vi "Overall Example.vi"() -> ()   [LabVIEW 2022 SP3]
uses:
  <instrlib>/openDAQ/Public/Classes/IInstance/IInstance.lvclass
  C:/Program Files (x86)/National Instruments/LabVIEW 2022/instr.lib/openDAQ/Public/Classes/IDevice/IDevice.lvclass
  C:/Program Files (x86)/National Instruments/LabVIEW 2022/instr.lib/openDAQ/Public/Classes/IComponent/IComponent.lvclass
  <instrlib>/openDAQ/Public/Classes/IComponent/IComponent.lvclass
  <instrlib>/openDAQ/Public/Classes/ISignal/ISignal.lvclass
  <instrlib>/openDAQ/Public/Classes/daqUtils/daqUtils.lvlib
  <instrlib>/openDAQ/Public/Classes/IDevice/IDevice.lvclass
panel:
  in  "btn:streamReader":bool
  in  "btn:multiReader":bool
  in  "btn:configureDevice":bool
  in  "Available Signals":i32[](listbox)
  in  "Btn:Stop":bool
  in  "MCL:available Devices":i32(listbox) caption="Available Devices"
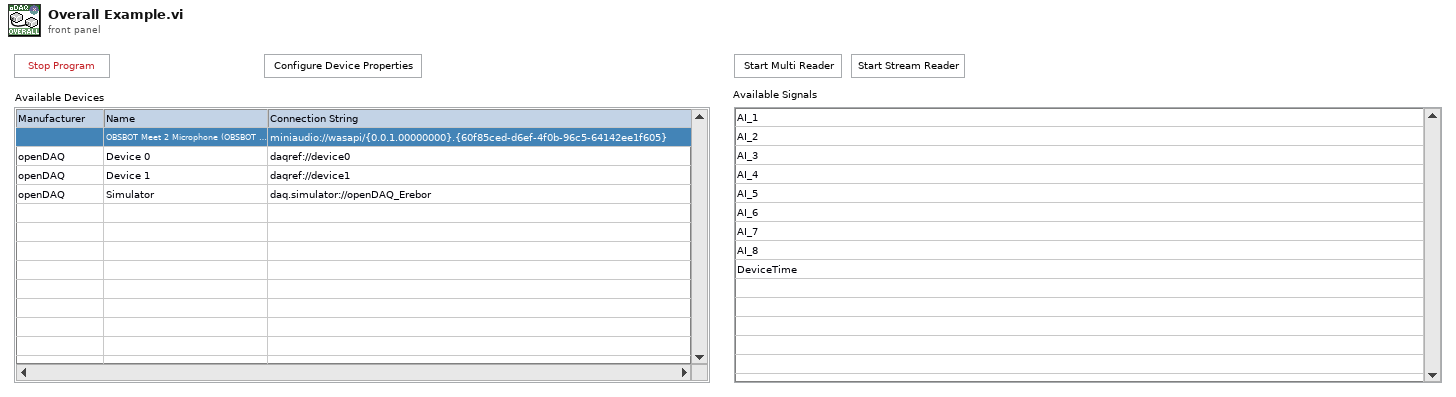
[diagram p1: front panel]
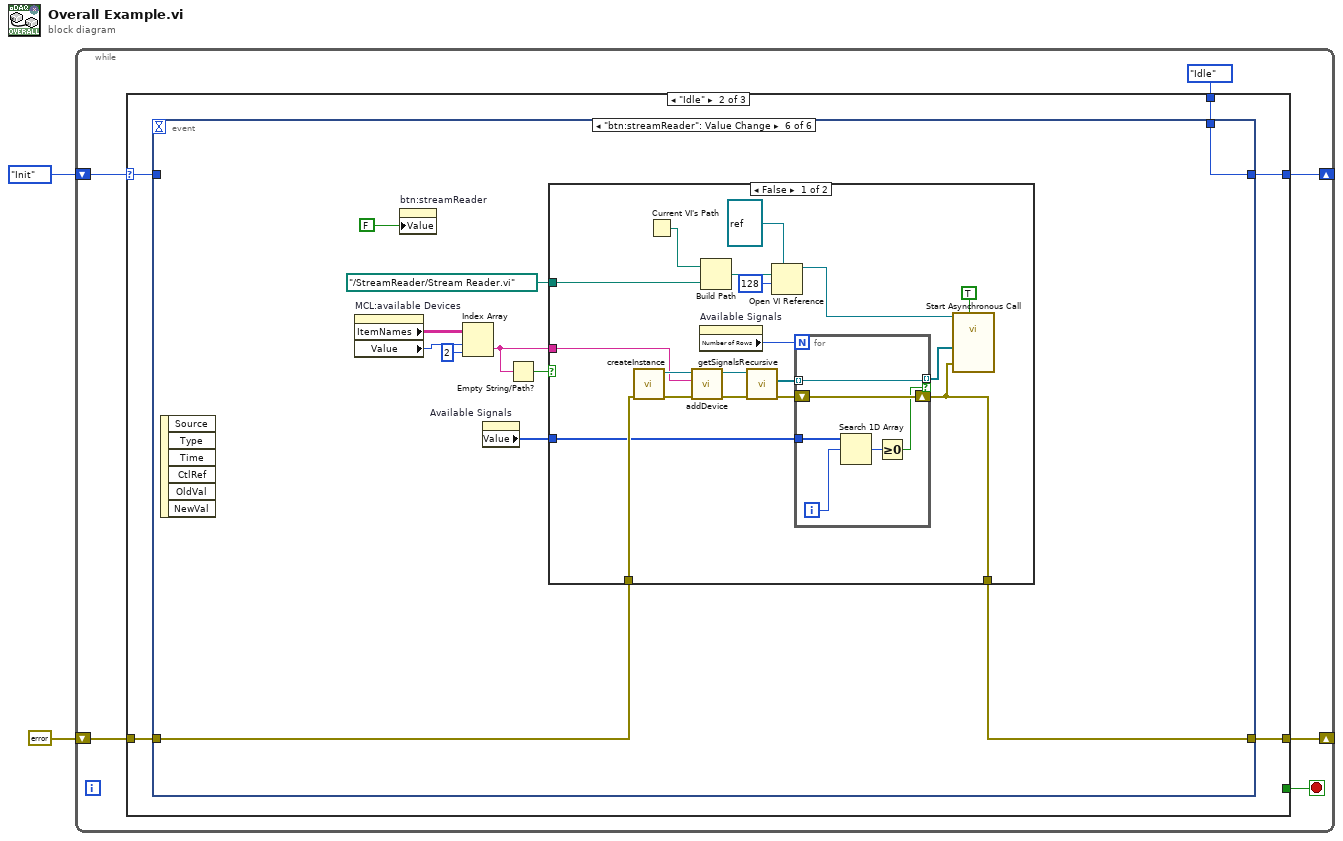
[diagram p0: block diagram]
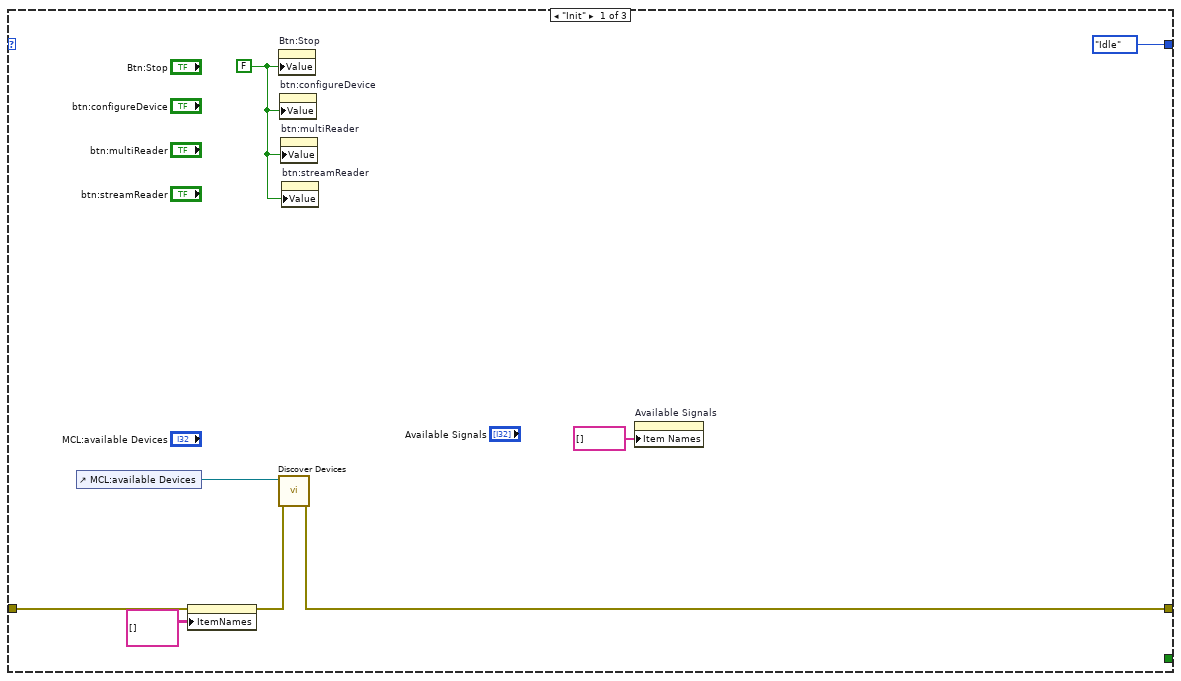
[diagram p2: hidden frame]
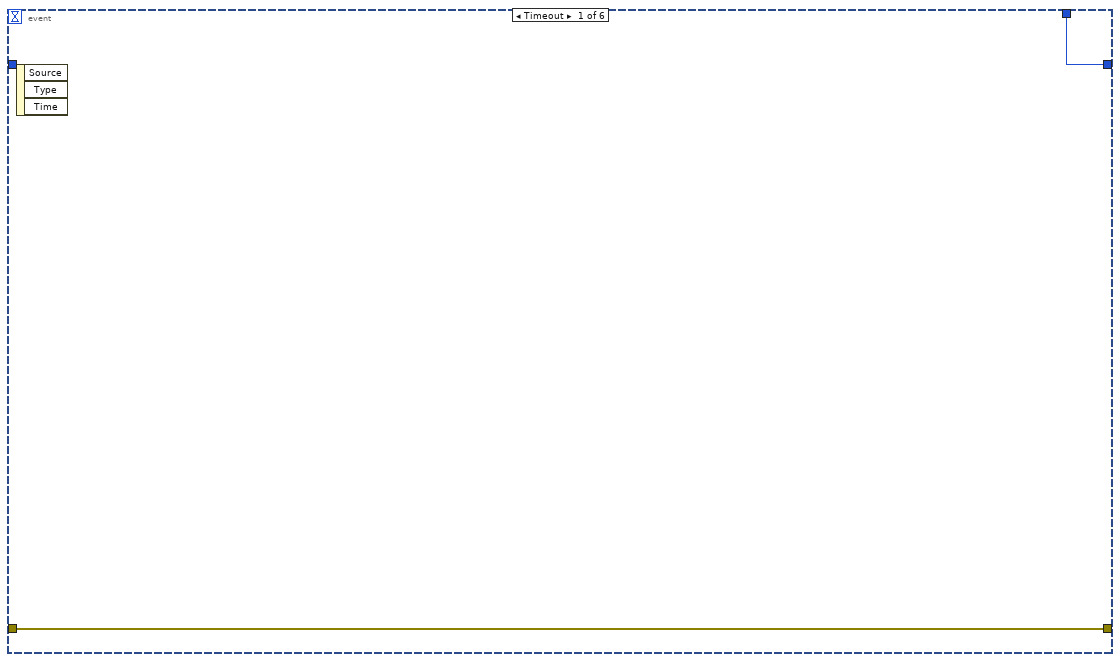
[diagram p3: hidden frame]
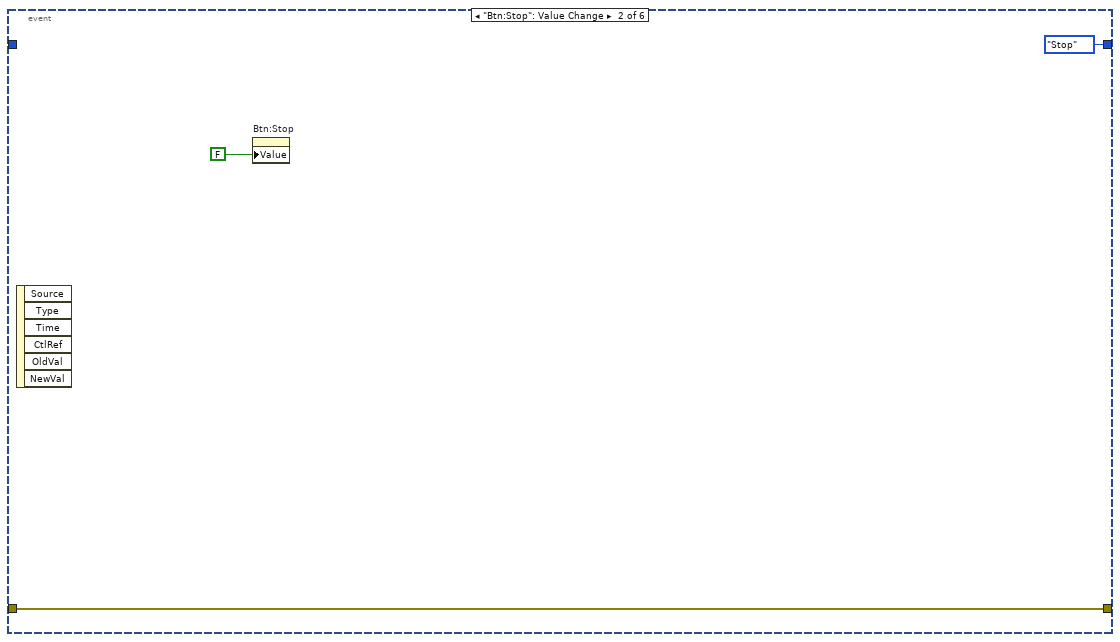
[diagram p4: hidden frame]
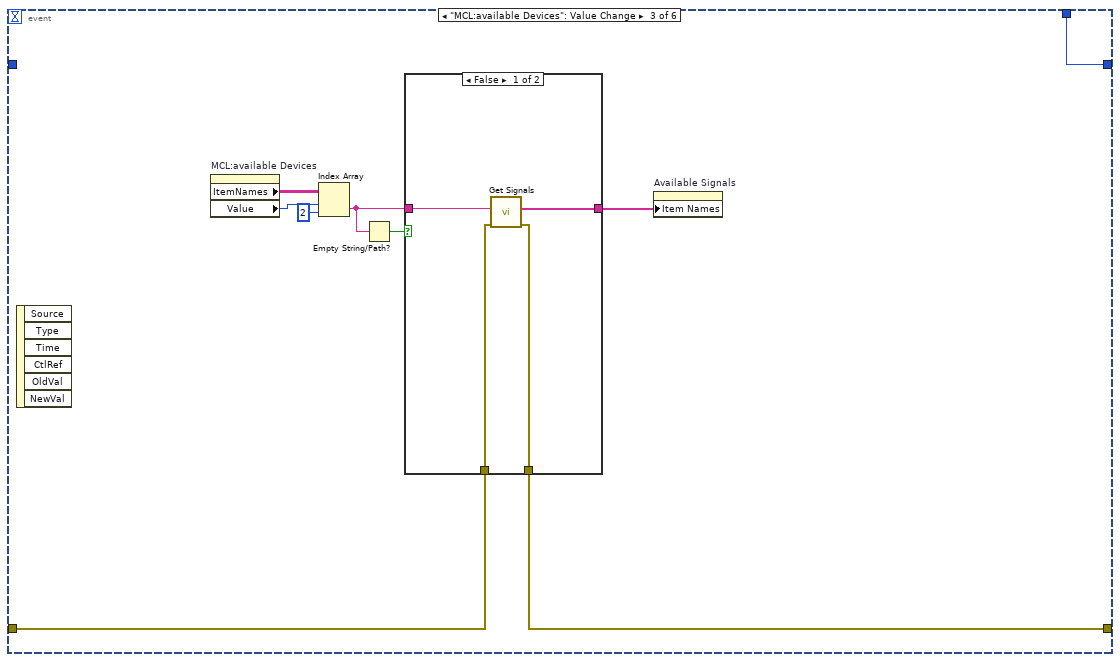
[diagram p5: hidden frame]
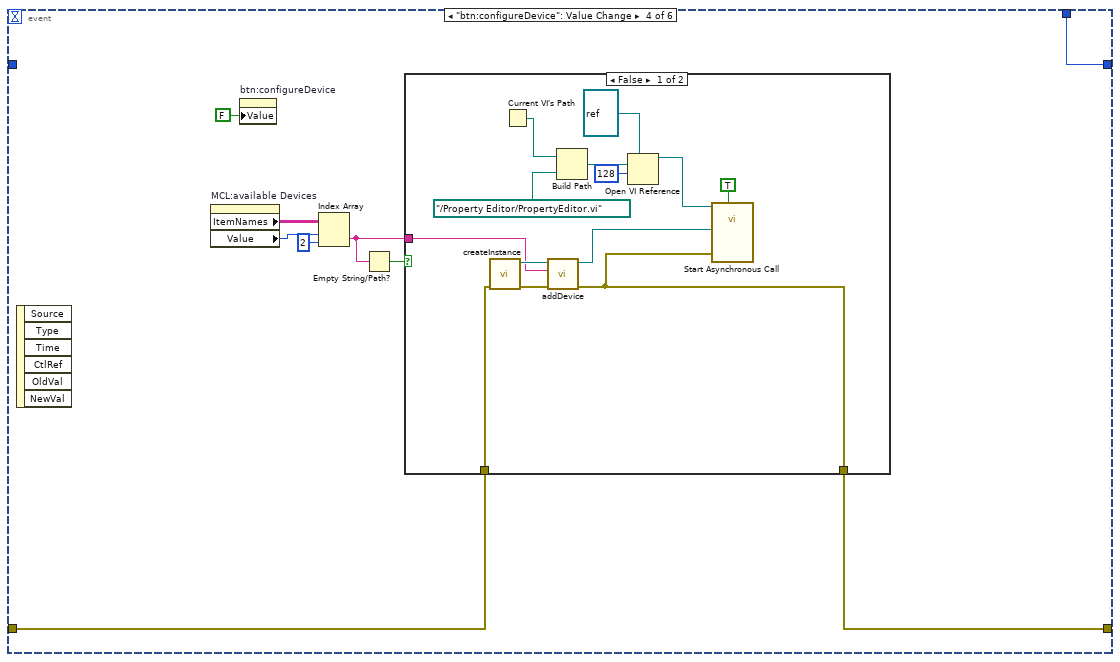
[diagram p7: hidden frame]
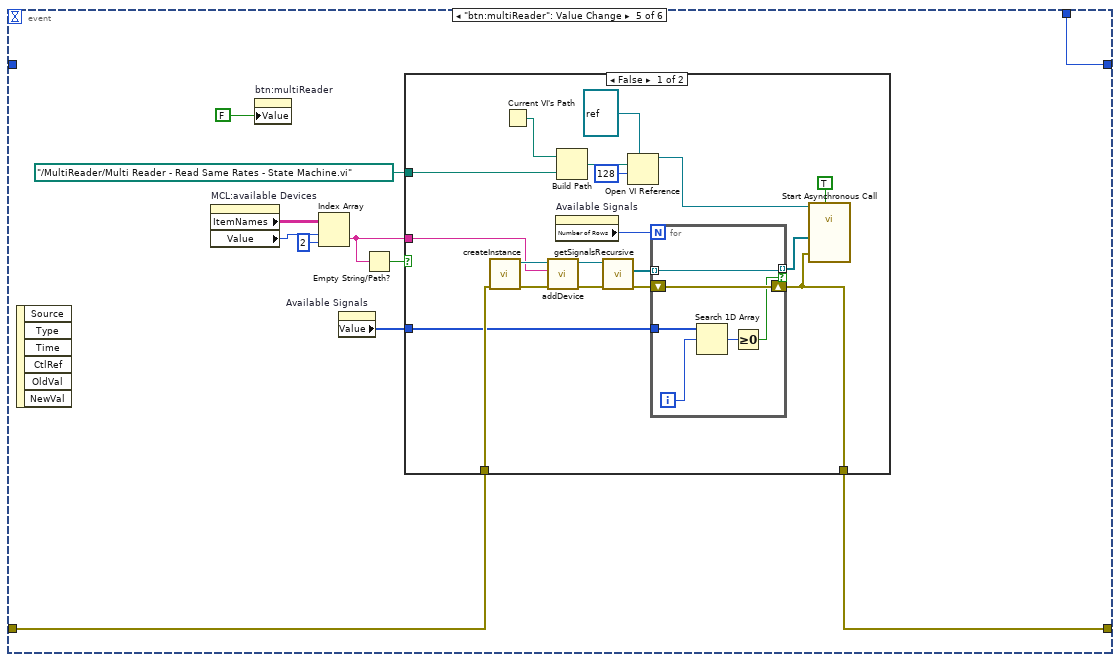
[diagram p9: hidden frame]
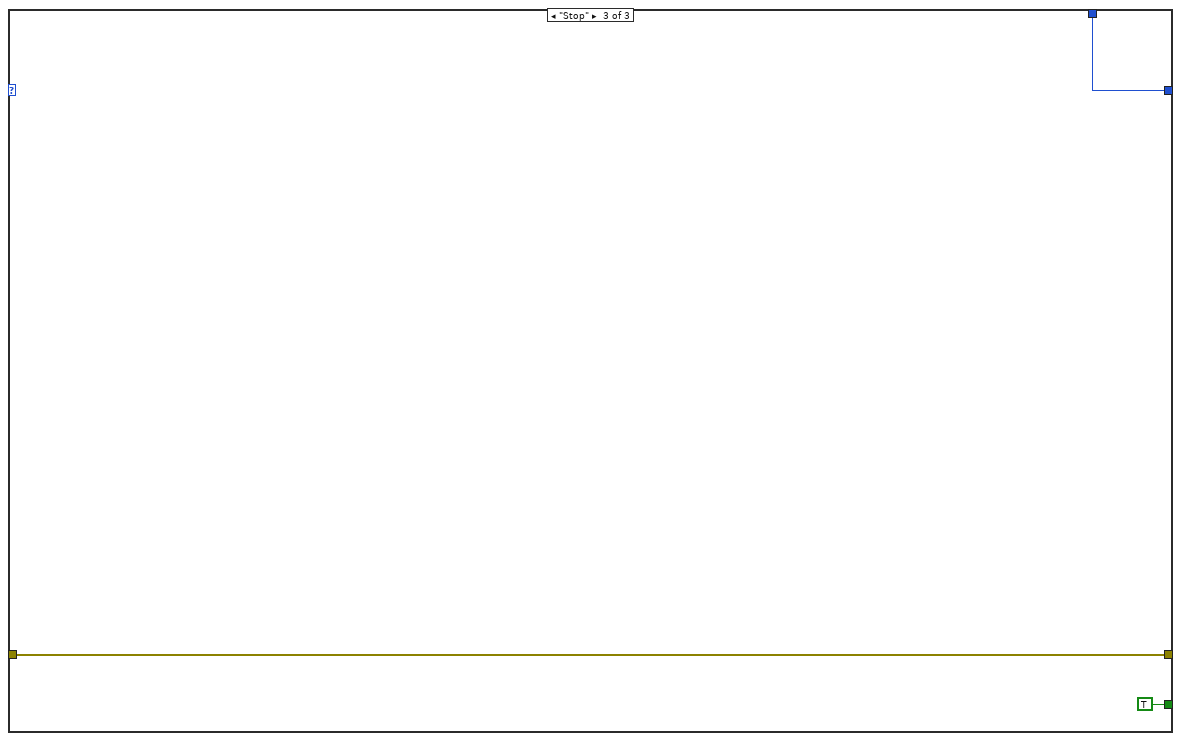
[diagram p12: hidden frame]
diagram:
  n1 = while {
    shift-right: [w7] -> _
    shift-left: enum16{"Init", "Idle", "Stop"}."Init" -> [w8]
    shift-right: [w5] -> _
    shift-left: errorcluster {"status"=FALSE, "code"=0, "source"=""} ("error constant") -> [w6]
    stop <- w3 stop-if-true
    n2 = case shown="\"Idle\"" w8 {
      selector: w8 -> [_ w21 _]
      tunnel: [enum16{"Init", "Idle", "Stop"}."Idle" w18 w140] -> w7
      tunnel: w6 -> [w13 w20 w139]
      tunnel: [w15 w19 w139] -> w5
      tunnel: enum16{"Init", "Idle", "Stop"}."Idle" -> [_ w17 w140]
      tunnel: [_ _ TRUE] -> w3
      frame "Init" {
        w9 = FALSE ("Btn:Stop")
        n3 = control-ref of="MCL:available Devices"() -> (w16:refnum<vi>)
        n4 = property on="MCL:available Devices" class="MCListbox (strict)"(error in=w13, "ItemNames"=string[][] [] ("Item Names")) -> (error out=w12:errorcluster)  [unwired: 1 in, 1 out]
        n5 = property on="Btn:Stop" class="Bool (strict)"("Value"=w9) -> ()  [unwired: 2 in, 2 out]
        n6 = call <instrlib>:"Discover Devices.vi"("error in (no error)"=w12, "Tree ref in"=w16) -> ("error out"=w15:errorcluster)  [unwired: 9 in]
        n7 = property on="btn:configureDevice" class="Bool (strict)"("Value"=w9) -> ()  [unwired: 2 in, 2 out]
        n8 = property on="btn:multiReader" class="Bool (strict)"("Value"=w9) -> ()  [unwired: 2 in, 2 out]
        n9 = property on="btn:streamReader" class="Bool (strict)"("Value"=w9) -> ()  [unwired: 2 in, 2 out]
        n10 = property on="Available Signals" class="LstBox (strict)"("Item Names"=string[] []) -> ()  [unwired: 2 in, 2 out]
      }
      frame "Idle" {
        n11 = event shown="[5] \"btn:streamReader\": Value Change" {
          selector: _ -> [_ _ _ _ _ _]
          dyn-events: _ -> [_ _ _ _ _ _]
          timeout: _ -> [_ _ _ _ _ _]
          tunnel: w21 -> [_ _ _ _ _ _]
          tunnel: w20 -> [w23 w24 w30 w44 w69 w106]
          tunnel: [w23 w24 w29 w43 w68 w105] -> w19
          tunnel: [w22 enum16{"Init", "Idle", "Stop"}."Stop" w27 w42 w67 w104] -> w18
          tunnel: w17 -> [w22 _ w27 w42 w67 w104]
          event Timeout {
            n12 = event-data() -> ()  [unwired: 1 in, 3 out]
          }
          event "Btn:Stop": Value Change {
            n13 = event-data() -> ()  [unwired: 1 in, 6 out]
            n14 = property on="Btn:Stop" class="Bool (strict)"("Value"=FALSE ("Btn:Stop")) -> ()  [unwired: 2 in, 2 out]
          }
          event "MCL:available Devices": Value Change {
            n15 = event-data() -> ()  [unwired: 1 in, 6 out]
            n16 = property on="MCL:available Devices" class="MCListbox (strict)"() -> ("ItemNames"=w35:string[][], "Value"=w34:i32)  [unwired: 2 in, 2 out]
            n17 = Index Array(array=w35, index (row)=w34, index (col)=2 ("disabled index (col)")) -> (element=w31:string)
            n18 = Empty String/Path?(string/path=w31) -> (empty?=w32:bool)
            n19 = case shown="False" w32 {
              tunnel: w31 -> [w39 _]
              tunnel: w30 -> [w38 w40]
              tunnel: [w37 w40] -> w29
              tunnel: [w36 _] -> w28
              frame False {
                n20 = call <instrlib>:"Get Signals.vi"("error in (no error)"=w38, "Connection String"=w39) -> ("error out"=w37:errorcluster, "Array"=w36:string[])  [unwired: 8 in]
              }
              frame True {
              }
            }
            n21 = property on="Available Signals" class="LstBox (strict)"("Item Names"=w28) -> ()  [unwired: 2 in, 2 out]
          }
          event "btn:configureDevice": Value Change {
            n22 = event-data() -> ()  [unwired: 1 in, 6 out]
            n23 = property on="MCL:available Devices" class="MCListbox (strict)"() -> ("ItemNames"=w49:string[][], "Value"=w48:i32)  [unwired: 2 in, 2 out]
            n24 = property on="btn:configureDevice" class="Bool (strict)"("Value"=FALSE ("btn:configureDevice")) -> ()  [unwired: 2 in, 2 out]
            n25 = Index Array(array=w49, index (row)=w48, index (col)=2 ("disabled index (col)")) -> (element=w45:string)
            n26 = Empty String/Path?(string/path=w45) -> (empty?=w46:bool)
            n27 = case shown="False" w46 {
              tunnel: w45 -> [w59 _]
              tunnel: w44 -> [w60 w63]
              tunnel: [w57 w63] -> w43
              frame False {
                n28 = call <instrlib>:"createInstance.vi"("error in (no error)"=w60) -> ("error out"=w61:errorcluster, "IInstance out"=w62:refnum<class "IInstance.lvclass">)  [unwired: 9 in]
                n29 = Current VI's Path() -> (path=w55:path)
                n30 = call <instrlib>:"addDevice.vi"("error in (no error)"=w61, "ConnectionString in"=w59, "IDevice in"=w62) -> ("error out"=w57:errorcluster, "IDevice out"=w58:refnum<class "IInstance.lvclass">)  [unwired: 6 in, 1 out]
                n31 = Build Path(base path=w55, name or relative path=path "../Property Editor/PropertyEditor.vi") -> (appended path=w56:path)
                n32 = Open VI Reference(type specifier VI Refnum (for type only)=refnum<vi> refnum, vi path=w56, options=128) -> (vi reference=w51:refnum<vi>)  [unwired: 3 in, 1 out]
                n33 = call-by-ref "Start Asynchronous Call"(reference=w51, "Popup? (F)"=TRUE, "error in (no error)"=w57, "Component in"=w58) -> ()  [unwired: 9 in, 3 out]
              }
              frame True {
              }
            }
          }
          event "btn:multiReader": Value Change {
            n34 = event-data() -> ()  [unwired: 1 in, 6 out]
            n35 = property on="MCL:available Devices" class="MCListbox (strict)"() -> ("ItemNames"=w74:string[][], "Value"=w73:i32)  [unwired: 2 in, 2 out]
            n36 = property on="btn:multiReader" class="Bool (strict)"("Value"=FALSE ("btn:configureDevice")) -> ()  [unwired: 2 in, 2 out]
            n37 = Index Array(array=w74, index (row)=w73, index (col)=2 ("disabled index (col)")) -> (element=w70:string)
            n38 = property on="Available Signals" class="LstBox (strict)"() -> ("Value"=w64:i32[])  [unwired: 2 in, 2 out]
            n39 = Empty String/Path?(string/path=w70) -> (empty?=w71:bool)
            n40 = case shown="False" w71 {
              tunnel: w70 -> [w90 _]
              tunnel: w69 -> [w91 w100]
              tunnel: [w80 w100] -> w68
              tunnel: path "../MultiReader/Multi Reader - Read Same Rates - State Machine.vi" ("name or relative path") -> [w84 _]
              tunnel: w64 -> [w78 _]
              frame False {
                n41 = call <instrlib>:"createInstance.vi"("error in (no error)"=w91) -> ("error out"=w92:errorcluster, "IInstance out"=w93:refnum<class "IInstance.lvclass">)  [unwired: 9 in]
                n42 = Current VI's Path() -> (path=w88:path)
                n43 = call <instrlib>:"addDevice.vi"("error in (no error)"=w92, "ConnectionString in"=w90, "IDevice in"=w93) -> ("error out"=w83:errorcluster, "IDevice out"=w82:refnum<class "IInstance.lvclass">)  [unwired: 6 in, 1 out]
                n44 = property on="Available Signals" class="LstBox (strict)"() -> ("Number of Rows"=w77:u32)  [unwired: 2 in, 2 out]
                n45 = Build Path(base path=w88, name or relative path=w84) -> (appended path=w89:path)
                n46 = call <instrlib>:"getSignalsRecursive.vi"("error in (no error)"=w83, "IDevice in"=w82) -> ("error out"=w79:errorcluster, "Available Sigals out"=w81:refnum<class "ISignal.lvclass">[])  [unwired: 7 in, 1 out]
                n47 = Open VI Reference(type specifier VI Refnum (for type only)=refnum<vi> refnum, vi path=w89, options=128) -> (vi reference=w85:refnum<vi>)  [unwired: 3 in, 1 out]
                n48 = for {
                  N: w77 -> [_]
                  tunnel: w81 -> [w98] mode=indexing
                  shift-right: [w99] -> w80
                  shift-left: w79 -> [w99]
                  tunnel: [w98] -> w76 mode=indexing if=w94
                  tunnel: w78 -> [w97]
                  i -> [w96]
                  n49 = Search 1D Array(1D array=w97, element=w96) -> (index of element=w95:i32)  [unwired: 1 in]
                  n50 = Greater Or Equal To 0?(x=w95) -> (x >= 0?=w94:bool)
                }
                n51 = call-by-ref "Start Asynchronous Call"(reference=w85, "Popup? (F)"=TRUE, "error in (no error)"=w80, "Signals in"=w76) -> ()  [unwired: 9 in, 3 out]
              }
              frame True {
              }
            }
          }
          event "btn:streamReader": Value Change {
            n52 = event-data() -> ()  [unwired: 1 in, 6 out]
            n53 = property on="MCL:available Devices" class="MCListbox (strict)"() -> ("ItemNames"=w111:string[][], "Value"=w110:i32)  [unwired: 2 in, 2 out]
            n54 = property on="btn:streamReader" class="Bool (strict)"("Value"=FALSE ("btn:configureDevice")) -> ()  [unwired: 2 in, 2 out]
            n55 = Index Array(array=w111, index (row)=w110, index (col)=2 ("disabled index (col)")) -> (element=w107:string)
            n56 = property on="Available Signals" class="LstBox (strict)"() -> ("Value"=w102:i32[])  [unwired: 2 in, 2 out]
            n57 = Empty String/Path?(string/path=w107) -> (empty?=w108:bool)
            n58 = case shown="False" w108 {
              tunnel: w107 -> [w127 _]
              tunnel: w106 -> [w128 w137]
              tunnel: [w117 w137] -> w105
              tunnel: path "../StreamReader/Stream Reader.vi" ("name or relative path") -> [w121 _]
              tunnel: w102 -> [w115 _]
              frame False {
                n59 = call <instrlib>:"createInstance.vi"("error in (no error)"=w128) -> ("error out"=w129:errorcluster, "IInstance out"=w130:refnum<class "IInstance.lvclass">)  [unwired: 9 in]
                n60 = Current VI's Path() -> (path=w125:path)
                n61 = call <instrlib>:"addDevice.vi"("error in (no error)"=w129, "ConnectionString in"=w127, "IDevice in"=w130) -> ("error out"=w120:errorcluster, "IDevice out"=w119:refnum<class "IInstance.lvclass">)  [unwired: 6 in, 1 out]
                n62 = property on="Available Signals" class="LstBox (strict)"() -> ("Number of Rows"=w114:u32)  [unwired: 2 in, 2 out]
                n63 = Build Path(base path=w125, name or relative path=w121) -> (appended path=w126:path)
                n64 = call <instrlib>:"getSignalsRecursive.vi"("error in (no error)"=w120, "IDevice in"=w119) -> ("error out"=w116:errorcluster, "Available Sigals out"=w118:refnum<class "ISignal.lvclass">[])  [unwired: 7 in, 1 out]
                n65 = Open VI Reference(type specifier VI Refnum (for type only)=refnum<vi> refnum, vi path=w126, options=128) -> (vi reference=w122:refnum<vi>)  [unwired: 3 in, 1 out]
                n66 = for {
                  N: w114 -> [_]
                  tunnel: w118 -> [w135] mode=indexing
                  shift-right: [w136] -> w117
                  shift-left: w116 -> [w136]
                  tunnel: [w135] -> w112 mode=indexing if=w131
                  tunnel: w115 -> [w134]
                  i -> [w133]
                  n67 = Search 1D Array(1D array=w134, element=w133) -> (index of element=w132:i32)  [unwired: 1 in]
                  n68 = Greater Or Equal To 0?(x=w132) -> (x >= 0?=w131:bool)
                }
                n69 = call-by-ref "Start Asynchronous Call"(reference=w122, "Popup? (F)"=TRUE, "error in (no error)"=w117, "Signals in"=w112) -> ()  [unwired: 9 in, 3 out]
              }
              frame True {
              }
            }
          }
        }
      }
      frame "Stop" {
      }
    }
  }
